vi "DribbleKick.vi"(1 "target gap":dbl[](array[numeric]), 4 "raio":dbl, 6 "target":dbl[](array[numeric]), 7 "firstCall?":bool, 8 "error in (no error)":errorcluster, 9 "Game":refnum<class "Game.lvclass">, 10 "Robot":refnum<class "Robot.lvclass">, 11 "KickToSkill in":refnum<class "KickToSkill.lvclass">) -> (0 "error out":errorcluster, 2 "Robot out":refnum<class "Robot.lvclass">, 3 "KickToSkill out":refnum<class "KickToSkill.lvclass">)   [LabVIEW 2024, in "KickToSkill.lvclass"]
uses:
  KickToSkill.lvclass
  Robot_class/Robot.lvclass
  C:/Users/as119/OneDrive/Documentos/roboIME/SSL_AI/Object_class/Object.lvclass
  Game_class/Game.lvclass
  DribbleKickStates.ctl
  Object_class/Object.lvclass/Object.ctl
  Robot_class/Robot.lvclass/Robot.ctl
  Game_class/Game.lvclass/Game.ctl
  <vilib>/Analysis/coordinate.llb/2D Cartesian Coordinate Rotation (Scalar).vi
  <vilib>/Analysis/_algsub.llb/Real Vector Norm.vi
  Game_class/Read NewParameters.vi
  Game_class/Read BallRef.vi
  Game_class/Read Parameters.lvclass.vi
  Object_class/Read position(x,y).vi
  Object_class/Read x.vi
  Object_class/Read y.vi
  Robot_class/Read orientation.vi
  Robot_class/Write dest_x_kick.vi
  Robot_class/Write dest_y_kick.vi
  Robot_class/Write dest_x.vi
  Robot_class/Write dest_y.vi
  Robot_class/Write dest_orientation.vi
  Ball_class/Ball.lvclass
  Parameters_class/Parameters.lvclass
  <vilib>/Analysis/NI_AALPro.lvlib
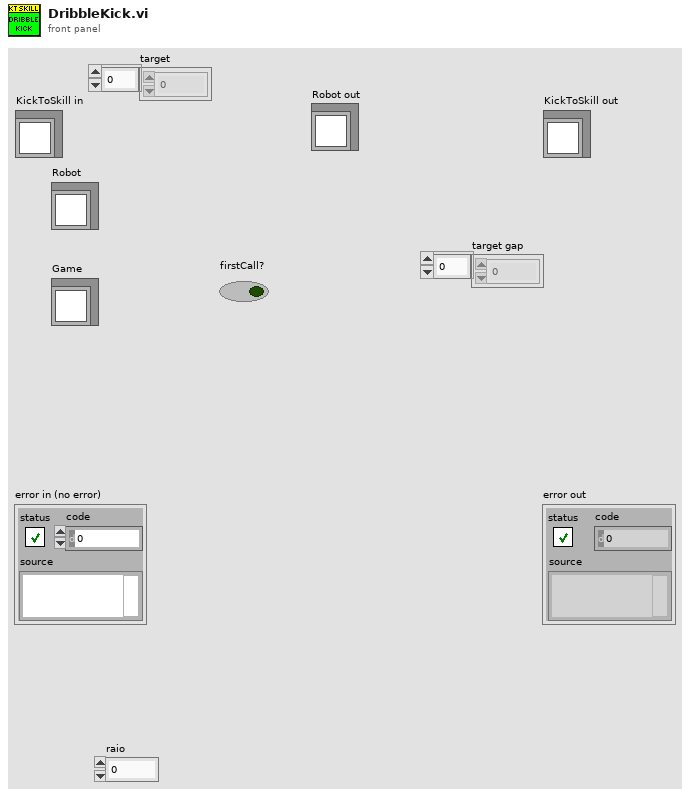
[diagram p1: front panel]
types:
  T1 = typedef "KickToSkill.lvclass/DribbleKickStates.ctl" = enum16{"aproximate", "turnDribbling", "kick"}
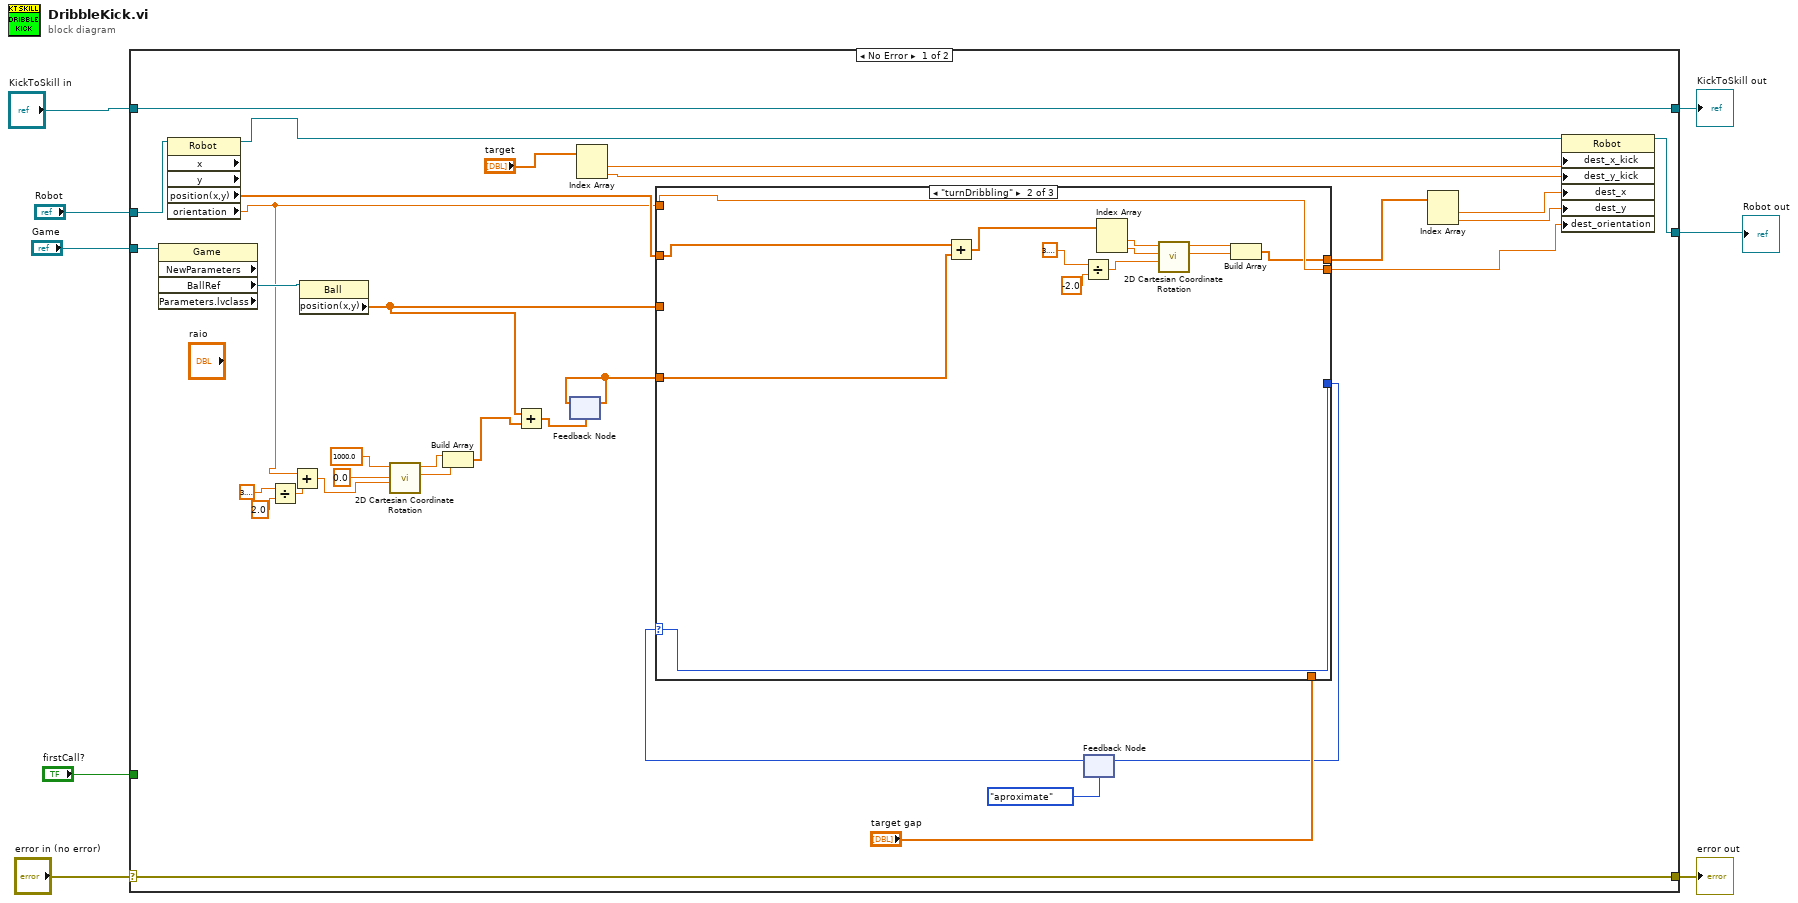
[diagram p0: block diagram]
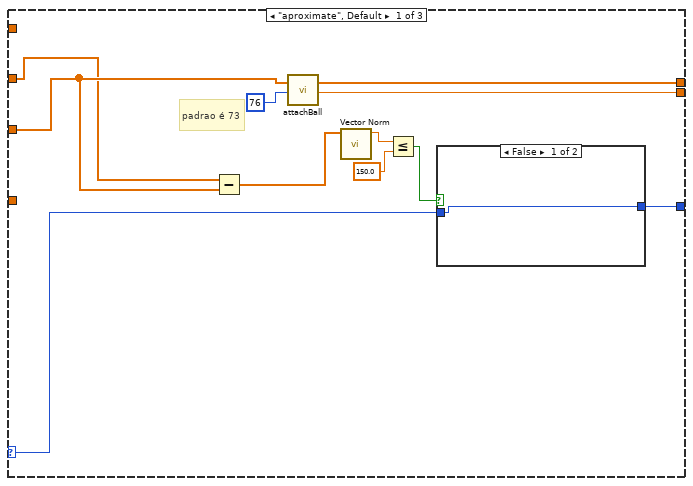
[diagram p2: hidden frame]
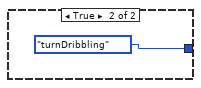
[diagram p3: hidden frame]
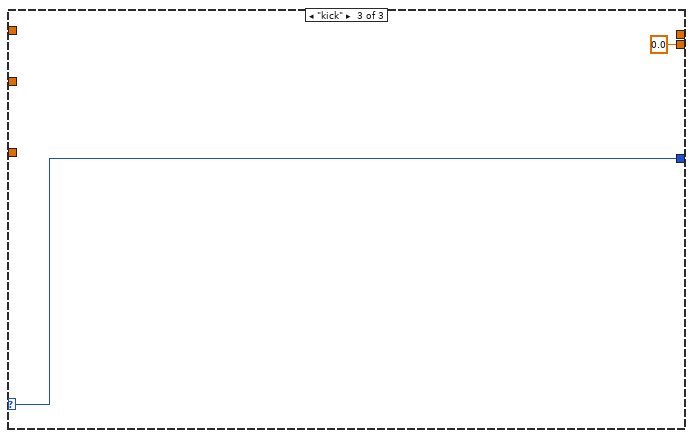
[diagram p4: hidden frame]
diagram:
  n1 = case shown="No Error" "error in (no error)" {
    selector: "error in (no error)" -> [w40 w71]
    tunnel: [w40 w71] -> w7
    tunnel: [w38 w70] -> w5
    tunnel: "KickToSkill in" -> [w38 w70]
    tunnel: "Robot" -> [w34 w69]
    tunnel: "Game" -> [w39 _]
    tunnel: [w37 w69] -> w2
    tunnel: "firstCall?" -> [_ _]
    frame No Error {
      n2 = property class="Game" props=["NewParameters", "BallRef", "Parameters.lvclass"](reference=w39) -> ("BallRef"=w35:refnum<class "Ball.lvclass">)  [unwired: 1 in, 4 out]
      n3 = property class="Robot" props=["x", "y", "position(x,y)", "orientation"](reference=w34) -> (reference out=w30:refnum<class "Robot.lvclass">, "position(x,y)"=w25:dbl[], "orientation"=w11:dbl)  [unwired: 1 in, 3 out]
      n4 = Divide(x=3.141592653589793, y=2.0) -> (x/y=w14:dbl)
      n5 = Add(x=w11, y=w14) -> (x+y=w15:dbl)
      n6 = property class="Ball"(reference=w35) -> ("position(x,y)"=w12:dbl[])  [unwired: 1 in, 2 out]
      n7 = call-poly <vilib>:"2D Cartesian Coordinate Rotation.vi"("theta"=w15, "y"=0.0 ("element"), "x"=1000.0 ("element")) -> ("y out"=w17:dbl, "x out"=w16:dbl)  [unwired: 6 in, 1 out]
      n8 = Build Array(w16, w17) -> (w13:dbl[])
      n9 = Add(x=w12, y=w13) -> (x+y=w10:dbl[])
      n10 = feedback #1(w10) -> (w9:dbl[])
      n11 = feedback-in #1(w9) -> ()
      n12 = Index Array(array="target") -> (element #1=w32:dbl, element #2=w31:dbl)  [unwired: 2 in]
      n13 = feedback #2(DribbleKickStates."aproximate" ("Enum")) -> (w27:T1)
      n14 = case shown="\"turnDribbling\"" w27 {
        selector: w27 -> [w43 w66 w67]
        tunnel: "target gap" -> [_ _ _]
        tunnel: w12 -> [w46 _ _]
        tunnel: [w51 w65 0.0 ("DestAngle")] -> w29
        tunnel: [w47 w66 w67] -> w28
        tunnel: w25 -> [w42 w64 _]
        tunnel: w11 -> [_ w65 _]
        tunnel: [w41 w57 _] -> w22
        tunnel: w9 -> [_ w54 _]
        frame "aproximate", Default {
          # "padrao é 73"
          n15 = Subtract(x=w42, y=w46) -> (x-y=w45:dbl[])
          n16 = call "attachBall.vi"("Dest"=w46, "Dist"=76) -> ("DestArray"=w41:dbl[], "DestAngle"=w51:dbl)  [unwired: 14 in, 2 out]
          n17 = call-poly <vilib>:"Vector Norm.vi"("Input Vector"=w45) -> ("norm"=w50:dbl)  [unwired: 9 in, 1 out]
          n18 = Less Or Equal?(x=w50, y=150.0) -> (x <= y?=w48:bool)
          n19 = case shown="False" w48 {
            tunnel: [w52 DribbleKickStates."turnDribbling" ("Enum")] -> w47
            tunnel: w43 -> [w52 _]
            frame False {
            }
            frame True {
            }
          }
        }
        frame "turnDribbling" {
          n20 = Add(x=w64, y=w54) -> (x+y=w55:dbl[])
          n21 = Divide(x=3.141592653589793, y=-2.0) -> (x/y=w62:dbl)
          n22 = Index Array(array=w55) -> (element #1=w61:dbl, element #2=w60:dbl)  [unwired: 2 in]
          n23 = call-poly <vilib>:"2D Cartesian Coordinate Rotation.vi"("theta"=w62, "y"=w60, "x"=w61) -> ("y out"=w58:dbl, "x out"=w59:dbl)  [unwired: 6 in, 1 out]
          n24 = Build Array(w59, w58) -> (w57:dbl[])
        }
        frame "kick" {
        }
      }
      n25 = feedback-in #2(w28) -> ()
      n26 = Index Array(array=w22) -> (element #1=w24:dbl, element #2=w23:dbl)  [unwired: 2 in]
      n27 = property class="Robot"(reference=w30, "dest_x_kick"=w32, "dest_y_kick"=w31, "dest_x"=w24, "dest_y"=w23, "dest_orientation"=w29) -> (reference out=w37:refnum<class "Robot.lvclass">)  [unwired: 1 in, 1 out]
    }
    frame Error {
    }
  }
  "error out" <- w7
  "KickToSkill out" <- w5
  "Robot out" <- w2
